vi "main.vi"() -> ()   [LabVIEW 2017]
panel:
  in  "stop":bool
  out "Result (ms)":dbl
  out "Message":string
  in  "Smash\nButton":bool
  out "indicator":bool
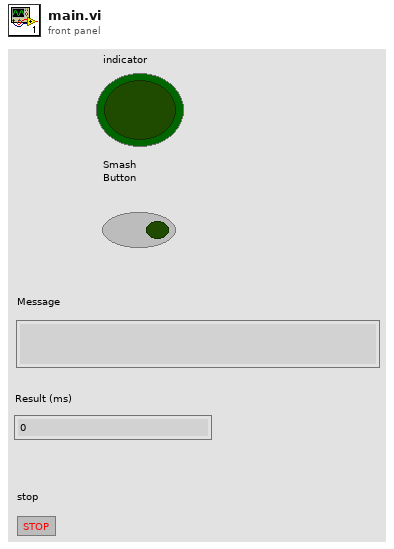
[diagram p1: front panel]
types:
  T1 = enum16{"BeginGame", "RandomWait", "WaiteForReaction", "CalculateResults"}
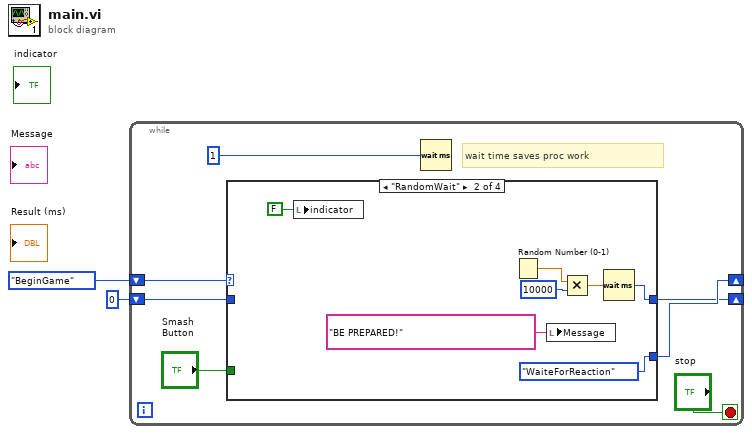
[diagram p0: block diagram]
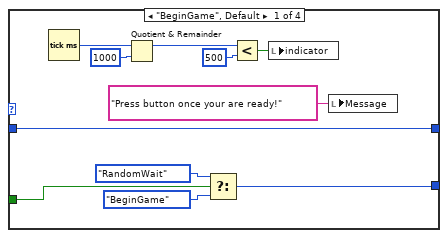
[diagram p2: hidden frame]
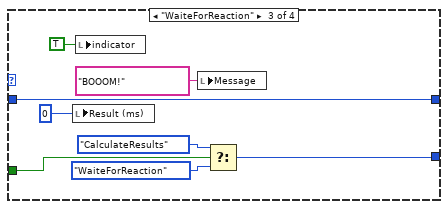
[diagram p3: hidden frame]
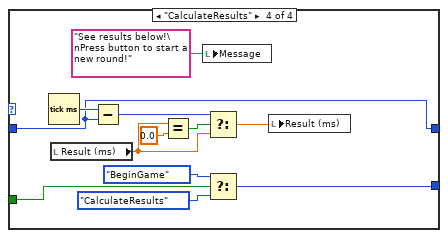
[diagram p4: hidden frame]
diagram:
  n1 = while {
    shift-right: [w6] -> _
    shift-left: T1."BeginGame" -> [w5]
    shift-right: [w4] -> _
    shift-left: 0 -> [w3]
    stop <- "stop" stop-if-true
    # "wait time saves proc work"
    n2 = case shown="\"RandomWait\"" w5 {
      tunnel: "Smash\nButton" -> [w14 _ w31 w45]
      tunnel: [w11 T1."WaiteForReaction" w30 w44] -> w6
      tunnel: [w10 w21 w29 w43] -> w4
      tunnel: w3 -> [w10 _ w29 w43]
      frame "BeginGame", Default {
        n3 = Tick Count (ms)() -> (millisecond timer value=w19:u32)
        n4 = Quotient & Remainder(x=w19, y=1000) -> (x-y*floor(x/y)=w16:u32)  [unwired: 1 out]
        n5 = Select(t=T1."RandomWait", s=w14, f=T1."BeginGame") -> (s? t:f=w11:T1)
        n6 = Less?(x=w16, y=500) -> (x < y?=w15:bool)
        n7 = local write "indicator"(w15) -> ()
        n8 = local write "Message"("Press button once your are ready!") -> ()
      }
      frame "RandomWait" {
        n9 = local write "indicator"(FALSE) -> ()
        n10 = Random Number (0-1)() -> (number: 0 to 1=w26:dbl)
        n11 = local write "Message"("BE PREPARED!") -> ()
        n12 = Multiply(x=w26, y=10000) -> (x*y=w22:dbl)
        n13 = Wait (ms)(milliseconds to wait=w22) -> (millisecond timer value=w21:u32)
      }
      frame "WaiteForReaction" {
        n14 = local write "Result (ms)"(0) -> ()
        n15 = local write "indicator"(TRUE) -> ()
        n16 = local write "Message"("BOOOM!") -> ()
        n17 = Select(t=T1."CalculateResults", s=w31, f=T1."WaiteForReaction") -> (s? t:f=w30:T1)
      }
      frame "CalculateResults" {
        n18 = Tick Count (ms)() -> (millisecond timer value=w46:u32)
        n19 = local read "Result (ms)"() -> (w36:dbl)
        n20 = Subtract(x=w46, y=w43) -> (x-y=w39:u32)
        n21 = Equal?(x=w36, y=0.0) -> (x = y?=w37:bool)
        n22 = local write "Message"("See results below!\nPress button to start a new round!") -> ()
        n23 = Select(t=w39, s=w37, f=w36) -> (s? t:f=w40:dbl)
        n24 = Select(t=T1."BeginGame", s=w45, f=T1."CalculateResults") -> (s? t:f=w44:T1)
        n25 = local write "Result (ms)"(w40) -> ()
      }
    }
    n26 = Wait (ms)(milliseconds to wait=u32 1) -> ()  [unwired: 1 out]
  }
